vi "d_posmatrix.vi"(1 "d-angle":dbl=0.04081632653061224 format="%.2f") -> (0 "d-matrix":dbl[][](array[numeric])=[[1.0, 0.0, 0.0, 0.0], [0.0, 1.0, 0.0, 0.0], [0.0, 0.0, 1.0, 0.0], [0.0, 0.0, 0.04081632653061224, 1.0]] format="%.2f")   [LabVIEW 2011]
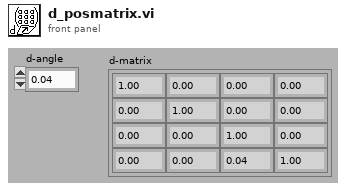
[diagram p1: front panel]
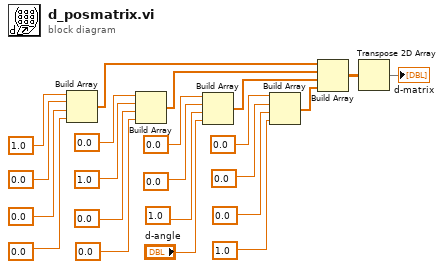
[diagram p0: block diagram]
diagram:
  n1 = Build Array(1.0, 0.0, 0.0, 0.0) -> (w20:dbl[])
  n2 = Build Array(0.0, 1.0, 0.0, 0.0) -> (w21:dbl[])
  n3 = Build Array(0.0, 0.0, 1.0, "d-angle") -> (w22:dbl[])
  n4 = Build Array(0.0, 0.0, 0.0, 1.0) -> (w17:dbl[])
  n5 = Build Array(w20, w21, w22, w17) -> (w4:dbl[][])
  n6 = Transpose 2D Array(2D array=w4) -> (transposed array=→"d-matrix":dbl[][])
